vi "ConAgent.vi"() -> ()   [LabVIEW 2022 SP3]
uses:
  <vilib>/Analysis/NI_AALPro.lvlib
  <vilib>/Utility/file.llb/Write To Spreadsheet File (DBL).vi
  <vilib>/Analysis/NI_AALBase.lvlib
  <vilib>/Analysis/baseanly.llb/Mean (DBL).vi
panel:
  in  "Save RMS?":bool
  in  "axis":u16(ring) items=["axis as count", "Axis as time (ms)", "Axis as distance (mm)"]
  out "flow velocity (cm/s)":dbl format="%.2f"
  in  "flow rate (ml/min)":dbl=8.0 format="%.2f"
  in  "tube diameter (cm)":dbl=0.3 format="%.4f"
  out "power spectrum of vertical yellow single line":cluster{i32, "df":dbl, dbl[]}(graph)
  out "mid freq of average":dbl format="%.2f"
  out "single frequency in ROI":dbl[](graph)
  out "Intensity Graph of power spectra in ROI":dbl[][](graph)
  out "RMS plot":cluster{i32, dbl, dbl[]}(graph)
  in  "Log scaling?":bool=TRUE
  in  "View Header?":bool
  out "Blow up of vertical blue Line":i16[](graph)
  in  "Header format":u16(ring) items=["Riverside Format", "Ron Linear"]
  out "Raw data":i16[][](graph)
  in  "new file path":path
  # "Select region to provide 3-D manipulation.\nKeep Yellow curser below and to left of blue."
  # "Horizontal yellow power spectra line"
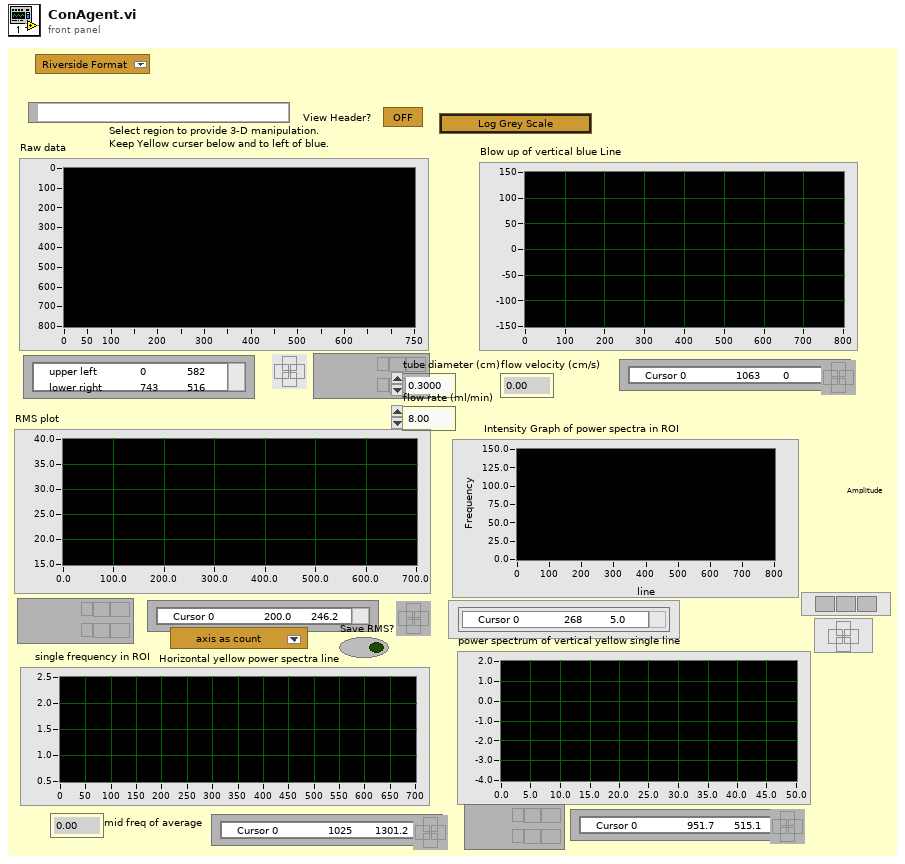
[diagram p1: front panel]
types:
  T1 = cluster{"Energy (microJ)":u8, "Damping (In Ohm)":u8, "HP Filt(KHz) ":u8, "LP Filt (MHz)":u8, "Gain (db)":u8, "prf (kHz)":sgl, "Distance between\nscan lines (mm)":u16, "Distance between\nscan planes (mm)":u16}
  T2 = cluster{"# rf points per line":u16, "# lines per scan":u16, "sample rate MHz":u16, "# A/D bits":u16, "# bytes per A/D":u16, "TGC Flag":u16, "A/D Type":string}
  T3 = cluster{"delay":sgl, "pivot distance":sgl, "sector scan angle":sgl, "operator":string, "Scan Mode":string, "location":string}
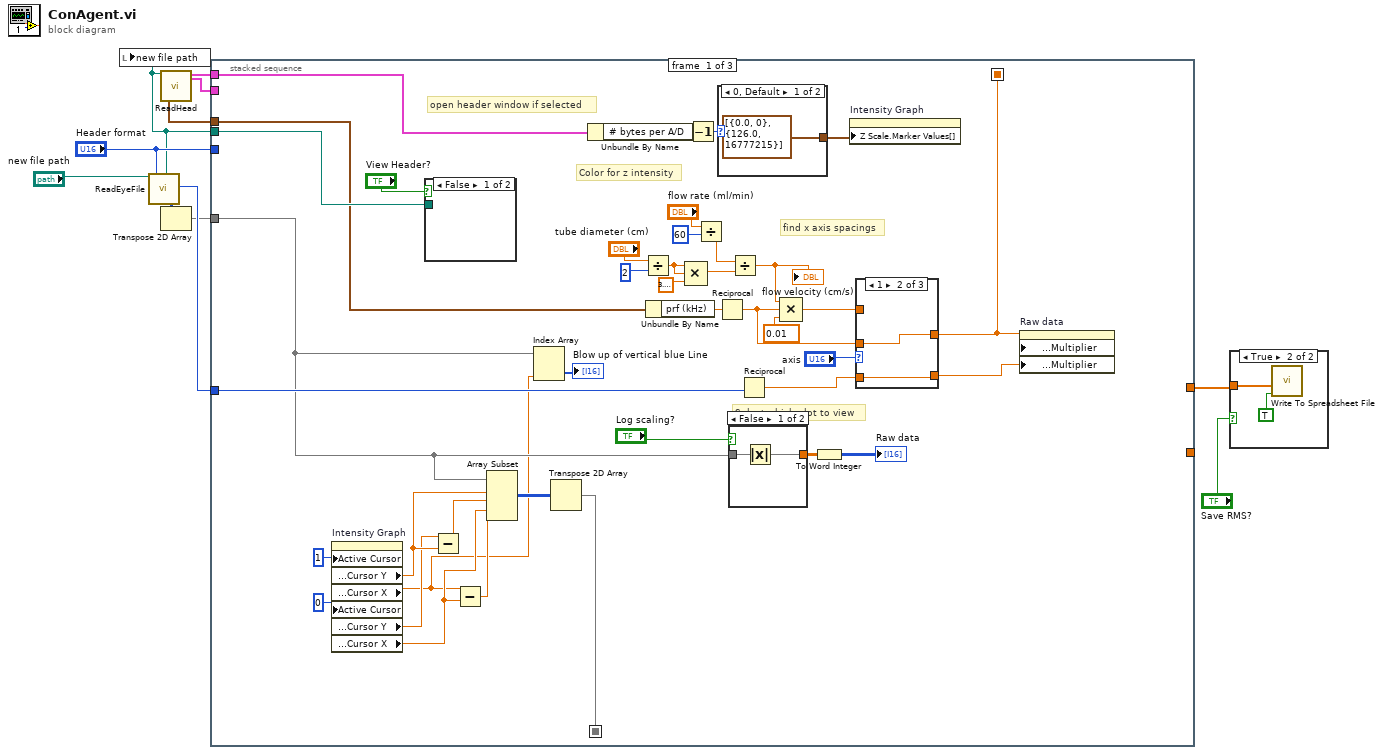
[diagram p0: block diagram]
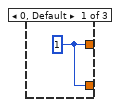
[diagram p3: hidden frame]
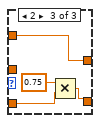
[diagram p4: hidden frame]
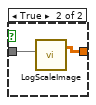
[diagram p5: hidden frame]
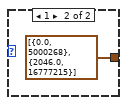
[diagram p6: hidden frame]
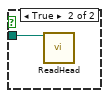
[diagram p7: hidden frame]
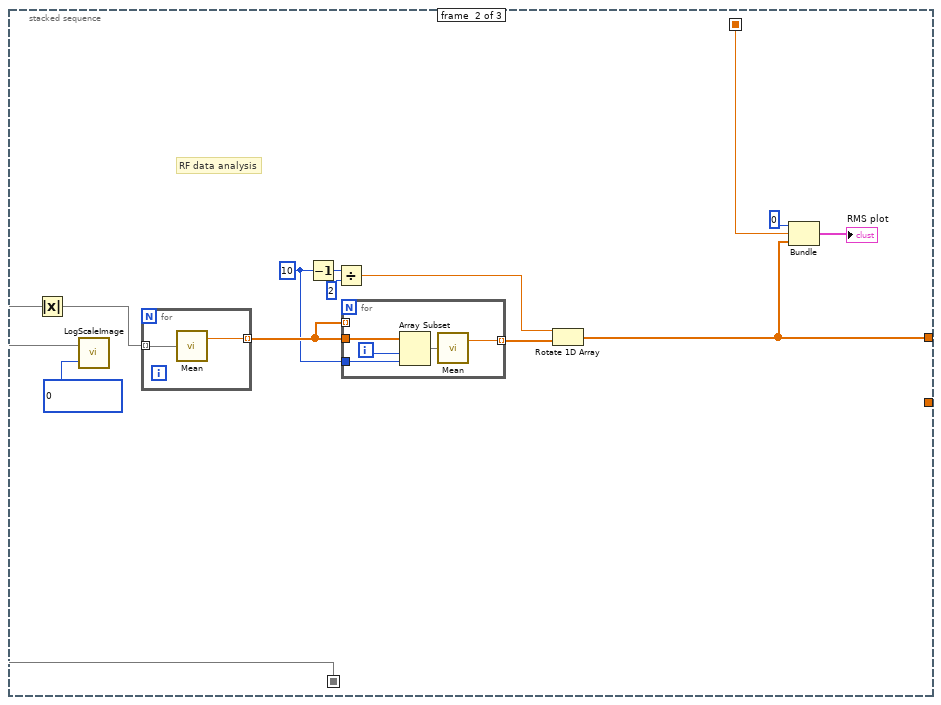
[diagram p8: hidden frame]
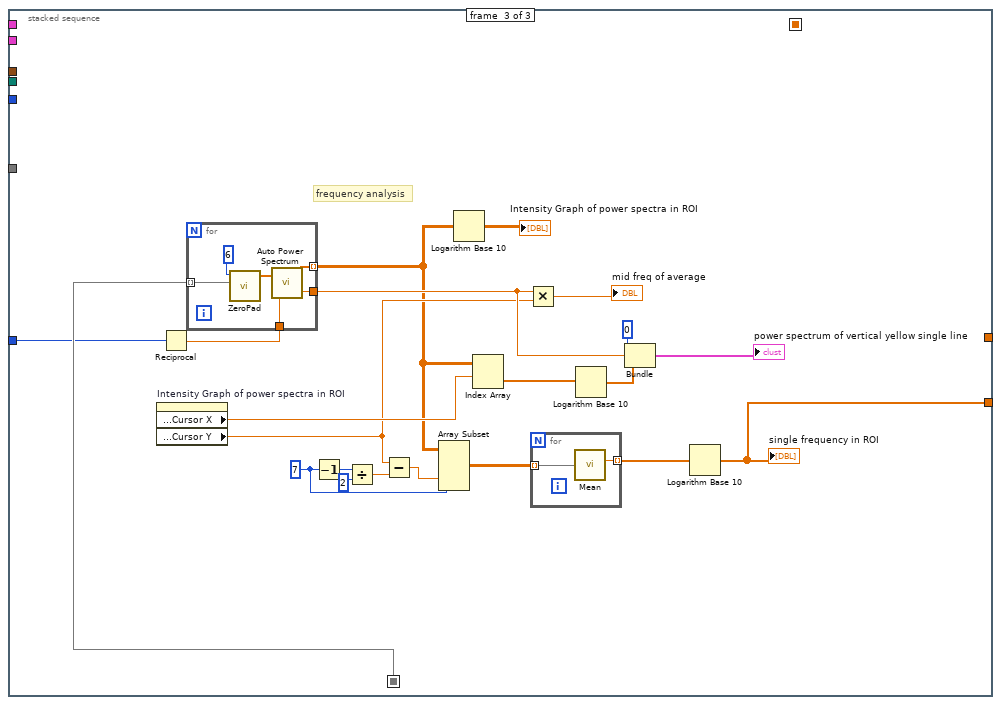
[diagram p9: hidden frame]
diagram:
  n1 = call "ReadEyeFile.vi"("new file path"="new file path", "Header format"="Header format") -> ("new path out"=w6:path, "2-D data array"=w9:i16[][], "sample rate MHz"=w10:u16)  [unwired: 15 out]
  n2 = local write "new file path"(w6) -> ()
  n3 = call "ReadHead.vi"("new file path"=w6) -> ("Pan Scan Settings"=w4:T1, "A/D info"=w5:T2, "Scan Info"=w11:T3)  [unwired: 16 out]
  n4 = Transpose 2D Array(2D array=w9) -> (transposed array=w1:i16[][])
  n5 = stacked-sequence {
    seq-local: [w34 _ _] -> [_ w70 w95]
    seq-local: [w18 _ _] -> [_ w73 _]
    tunnel: w11 -> [_ _ _]
    tunnel: w10 -> [w16 _ w90]
    tunnel: w1 -> [w14 _ _]
    tunnel: "Header format" -> [_ _ _]
    tunnel: w6 -> [w35 _ _]
    tunnel: w5 -> [w49 _ _]
    tunnel: w4 -> [w19 _ _]
    tunnel: [_ w67 _] -> w2
    tunnel: [_ _ w88] -> _
    frame #0 {
      # "find x axis spacings"
      # "Color for z intensity"
      # "open header window if selected"
      # "Select which plot to view"
      n6 = property on="Intensity Graph" class="IntGraph (strict)"("Active Cursor"=u32 1 ("Write Attribute"), "Active Cursor"=u32 0 ("Write Attribute")) -> ("Cursor.Cursor Position:Cursor Y"=w37:dbl, "Cursor.Cursor Position:Cursor X"=w12:dbl, "Cursor.Cursor Position:Cursor Y"=w36:dbl, "Cursor.Cursor Position:Cursor X"=w41:dbl)  [unwired: 2 in, 2 out]
      n7 = case shown="False" "View Header?" {
        tunnel: w35 -> [_ w65]
        frame False {
        }
        frame True {
          n8 = call "ReadHead.vi"("new file path"=w65) -> ()  [unwired: 19 out]
        }
      }
      n9 = Subtract(x=w36, y=w37) -> (x-y=w43:dbl)
      n10 = Subtract(x=w12, y=w41) -> (x-y=w42:dbl)
      n11 = Array Subset(array=w14, index (row)=w37, length (row)=w43, index (col)=w41, length (col)=w42) -> (w38:i16[][])
      n12 = Index Array(array=w14, index (col)=w12) -> (element=→"Blow up of vertical blue Line":i16[])  [unwired: 1 in]
      n13 = Transpose 2D Array(2D array=w38) -> (transposed array=w34:i16[][])
      n14 = Unbundle By Name(w49) -> ("# bytes per A/D"=w48:u16)
      n15 = Divide(x="tube diameter (cm)", y=2) -> (x/y=w30:dbl)
      n16 = Unbundle By Name(w19) -> ("prf (kHz)"=w32:sgl)
      n17 = Compound Arithmetic op=MULTIPLY(w30, w30, 3.141592653589793) -> (w26:dbl)
      n18 = Decrement(x=w48) -> (x-1=w47:u16)
      n19 = Divide(x="flow rate (ml/min)", y=60) -> (x/y=w25:dbl)
      n20 = Reciprocal(x=w32) -> (1/x=w21:sgl)
      n21 = case shown="0, Default" w47 {
        tunnel: [cluster{dbl, u32}[] [{0.0, 0}, {126.0, 16777215}] ("color scheme 3") cluster{dbl, u32}[] [{0.0, 5000268}, {2046.0, 16777215}] ("color scheme 3")] -> w50
        frame 0, Default {
        }
        frame 1 {
        }
      }
      n22 = case shown="False" "Log scaling?" {
        tunnel: [w59 w62] -> w46
        tunnel: w14 -> [w60 w61]
        frame False {
          n23 = Absolute Value(x=w60) -> (abs(x)=w59:i16[][])
        }
        frame True {
          n24 = call "LogScaleImage.vi"("input array"=w61) -> ("log scale image"=w62:dbl[][])  [unwired: 1 in, 1 out]
        }
      }
      n25 = Divide(x=w25, y=w26) -> (x/y=w24:dbl)
      "flow velocity (cm/s)" <- w24
      n26 = Reciprocal(x=w16) -> (1/x=w15:dbl)
      n27 = Compound Arithmetic op=MULTIPLY(w24, w21, 0.01) -> (w20:dbl)
      n28 = To Word Integer(number=w46) -> (16bit integer=→"Raw data":i16[][])
      n29 = property on="Intensity Graph" class="IntGraph (strict)"("Z Scale.Marker Values[]"=w50) -> ()  [unwired: 2 in, 2 out]
      n30 = case shown="1" "axis" {
        tunnel: [w52 w54 w58] -> w18
        tunnel: w21 -> [_ w54 _]
        tunnel: w20 -> [_ _ w58]
        tunnel: [w52 w53 w57] -> w17
        tunnel: w15 -> [_ w53 w55]
        frame 0, Default {
          w52 = 1
        }
        frame 1 {
        }
        frame 2 {
          n31 = Multiply(x=0.75, y=w55) -> (x*y=w57:dbl)
        }
      }
      n32 = property on="Raw data" class="IntGraph (strict)"("X Scale.Offset and Multiplier:Multiplier"=w18, "Y Scale.Offset and Multiplier:Multiplier"=w17) -> ()  [unwired: 2 in, 2 out]
    }
    frame #1 {
      w69 = 10
      # "RF data analysis"
      n33 = Absolute Value(x=w70) -> (abs(x)=w68:i16[][])
      n34 = call "LogScaleImage.vi"("A/D bits"=u16 0 ("bytes"), "input array"=w70) -> ()  [unwired: 2 out]
      n35 = for {
        tunnel: w68 -> [w84] mode=indexing
        tunnel: [w85] -> w71 mode=indexing
        n36 = call-poly <vilib>:"Mean.vi"("X"=w84) -> ("mean"=w85:dbl)  [unwired: 1 out]
      }
      n37 = Decrement(x=w69) -> (x-1=w75:i32)
      n38 = Divide(x=w75, y=2) -> (x/y=w74:dbl)
      n39 = for {
        tunnel: w71 -> [w83]
        tunnel: w69 -> [w81]
        tunnel: w71 -> [_] mode=indexing
        tunnel: [w79] -> w66 mode=indexing
        i -> [w82]
        n40 = Array Subset(array=w83, index=w82, length=w81) -> (w80:dbl[])
        n41 = call-poly <vilib>:"Mean.vi"("X"=w80) -> ("mean"=w79:dbl)  [unwired: 1 out]
      }
      n42 = Rotate 1D Array(1:w66, 2:w74) -> (0:w67:dbl[])
      n43 = Bundle(0, w73, w67) -> (→"RMS plot":cluster{i32, dbl, dbl[]})  [unwired: 1 out]
    }
    frame #2 {
      w100 = 7
      # "frequency analysis"
      n44 = property on="Intensity Graph of power spectra in ROI" class="IntGraph (strict)"() -> ("Cursor.Cursor Position:Cursor X"=w91:dbl, "Cursor.Cursor Position:Cursor Y"=w89:dbl)  [unwired: 2 in, 2 out]
      n45 = Reciprocal(x=w90) -> (1/x=w97:dbl)
      n46 = for {
        tunnel: w95 -> [w109] mode=indexing
        tunnel: w97 -> [w112]
        tunnel: [w111] -> w87 mode=indexing
        tunnel: [w110] -> w98
        n47 = call "ZeroPad.vi"("Input Array"=w109, "FFT size"=6) -> ("Ouput Array"=w114:dbl[])  [unwired: 4 out]
        n48 = call <vilib>:"Auto Power Spectrum.vi"("dt"=w112, "Signal (V)"=w114) -> ("df"=w110:dbl, "Power Spectrum (V^2 rms)"=w111:dbl[])
      }
      n49 = Decrement(x=w100) -> (x-1=w104:i32)
      n50 = Divide(x=w104, y=2) -> (x/y=w103:dbl)
      n51 = Subtract(x=w89, y=w103) -> (x-y=w102:dbl)
      n52 = Array Subset(array=w87, index (col)=w102, length (col)=w100) -> (w101:dbl[][])  [unwired: 2 in]
      n53 = Logarithm Base 10(1:w87) -> (0:→"Intensity Graph of power spectra in ROI":dbl[][])
      n54 = Index Array(array=w87, index (row)=w91) -> (element=w96:dbl[])  [unwired: 1 in]
      n55 = Multiply(x=w98, y=w89) -> (x*y=→"mid freq of average":dbl)
      n56 = for {
        tunnel: [w108] -> w106 mode=indexing
        tunnel: w101 -> [w107] mode=indexing
        n57 = call-poly <vilib>:"Mean.vi"("X"=w107) -> ("mean"=w108:dbl)  [unwired: 1 out]
      }
      n58 = Logarithm Base 10(1:w96) -> (0:w92:dbl[])
      n59 = Bundle(0, "df"=w98, w92) -> (→"power spectrum of vertical yellow single line":cluster{i32, "df":dbl, dbl[]})  [unwired: 1 out]
      n60 = Logarithm Base 10(1:w106) -> (0:w88:dbl[])
      "single frequency in ROI" <- w88
    }
  }
  n61 = case shown="True" "Save RMS?" {
    tunnel: w2 -> [_ w116]
    frame False {
    }
    frame True {
      n62 = call-poly <vilib>:"Write To Spreadsheet File.vi"("append to file? (new file:F)"=TRUE, "1D data"=w116) -> ()  [unwired: 4 in, 3 out]
    }
  }
